vi "Initialize.vi"(8 "error in (no error)":errorcluster, 11 "RS232 to GPIB ConvBox in":refnum<class "RS-xxx to GPIB ConvBox.lvclass">) -> (0 "error out":errorcluster, 3 "RS232 to GPIB ConvBox out":refnum<class "RS-xxx to GPIB ConvBox.lvclass">)   [LabVIEW 2019, in "Protocols.lvlib" / "RS-xxx to GPIB ConvBox.lvclass"]
uses:
  RS-xxx to GPIB ConvBox.lvclass
  RS-xxx to GPIB ConvBox.lvclass/RS-xxx to GPIB ConvBox.ctl
  Data Access/Read IST bit sense.vi
  Data Access/Read Port.vi
  Data Access/Read ConvBox Address.vi
  Data Access/Read Assert Ren with IFC.vi
  Data Access/Read System controller.vi
  Data Access/Write Port Ref.vi
  <vilib>/Utility/error.llb/Error Cluster From Error Code.vi
  Protocol Parent/Protocol Parent.lvclass
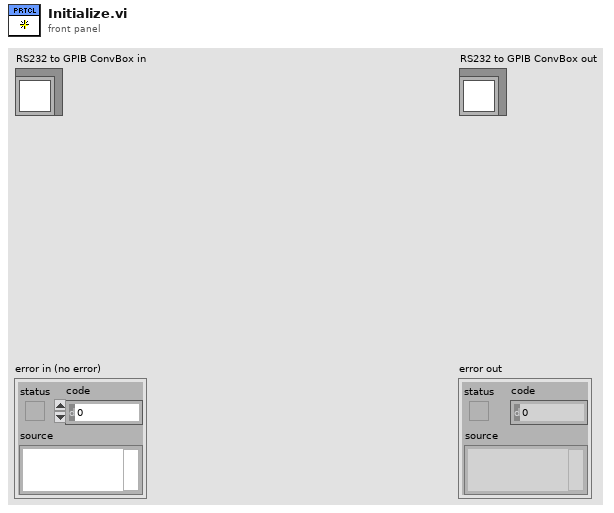
[diagram p1: front panel]
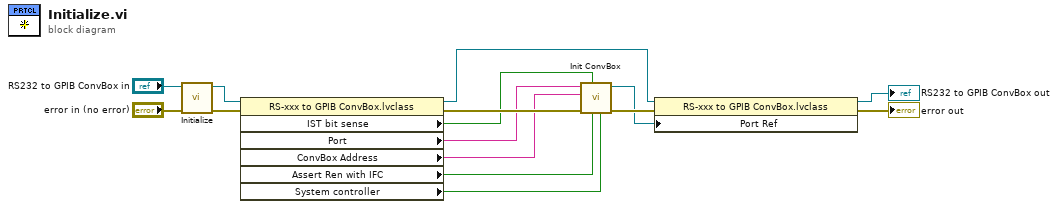
[diagram p0: block diagram]
diagram:
  n1 = call-parent "Initialize.vi"("error in (no error)"="error in (no error)", "Protocol Parent in"="RS232 to GPIB ConvBox in") -> ("error out"=w12:errorcluster, "Protocol Parent out"=w13:refnum<class "RS-xxx to GPIB ConvBox.lvclass">)  [unwired: 8 in]
  n2 = property class="RS-xxx to GPIB ConvBox.lvclass"(reference=w13, error in=w12) -> (reference out=w5:refnum<class "RS-xxx to GPIB ConvBox.lvclass">, error out=w11:errorcluster, "IST bit sense"=w8:bool, "Port"=w9:string, "ConvBox Address"=w10:string, "Assert Ren with IFC"=w7:bool, "System controller"=w6:bool)
  n3 = call "Init ConvBox.vi"("system controller (T)"=w6, "Assert Ren with IFC"=w7, "IST bit sense (T)"=w8, "error in (no error)"=w11, "Address"=w10, "Serial Port"=w9) -> ("error out"=w4:errorcluster, "Serial Port Out"=w1:refnum<visa-resource-name>)  [unwired: 4 in]
  n4 = property class="RS-xxx to GPIB ConvBox.lvclass"(reference=w5, error in=w4, "Port Ref"=w1) -> (reference out=→"RS232 to GPIB ConvBox out":refnum<class "RS-xxx to GPIB ConvBox.lvclass">, error out=→"error out":errorcluster)
